vi "Autonomous Independent.vi"   [LabVIEW 2018]
doc: "This VI is called when autonomous begins, and will automatically be terminated when autonomous ends. You can carry out timed or sensor driven robot movement independently without needing to return to the caller."
uses:
  RobotGlobal.vi
  Classes/Pnematics control/Pneumatics.lvclass
  Classes/Pnematics control/Solenoids/Solenoids.lvclass
panel:
  # "Be sure to right-click and choose Data Operations>>Make Current Value default if you want to save the array values with the VI"
types:
  T1 = typedef "RobotObjects.ctl" = cluster{"Drive.lvclass":refnum<class "Drive.lvclass">, "Pneumatics.lvclass":refnum<class "Pneumatics.lvclass">, "Vision.lvclass":refnum<class "Vision.lvclass">, "Joysticks.lvclass":refnum<class "Joysticks.lvclass">, "Elevator.lvclass":refnum<class "Elevator.lvclass">, "Hatch.lvclass":refnum<class "Hatch.lvclass">, "Cargo.lvclass":refnum<class "Cargo.lvclass">}
  T2 = typedef "Pneumatics control.lvlib/Pneumatics.lvclass/Solenoids.ctl" = cluster{"DriveShift":refnum<class "Solenoids.lvclass">, "ArmLock":refnum<class "Solenoids.lvclass">, "HatchArm":refnum<class "Solenoids.lvclass">, "HatchGrabber":refnum<class "Solenoids.lvclass">}
  T3 = cluster{"[0]":refnum<class "Solenoids.lvclass">, "[1]":refnum<class "Solenoids.lvclass">, "[2]":refnum<class "Solenoids.lvclass">, "[3]":refnum<class "Solenoids.lvclass">}
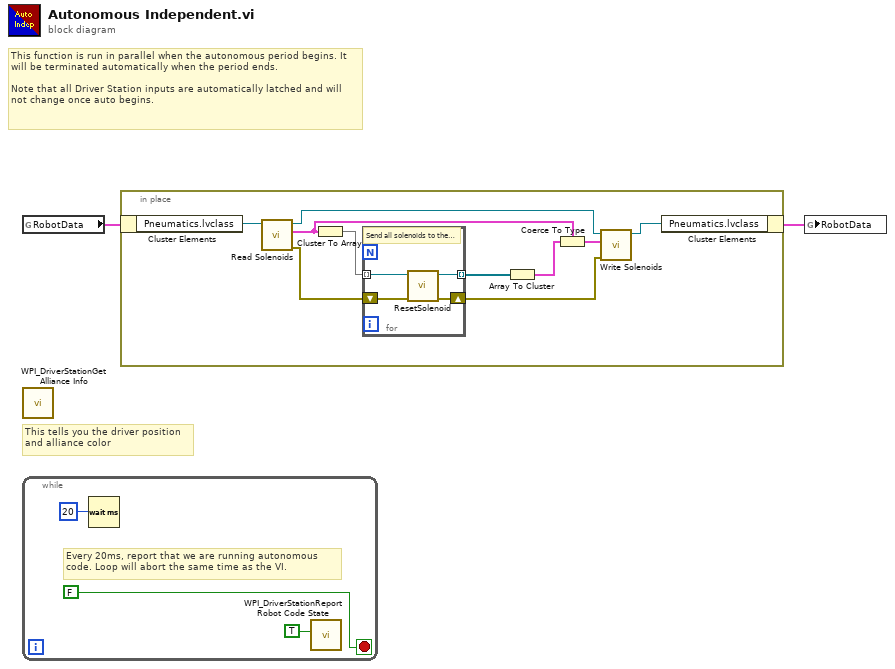
[diagram p0: block diagram]
diagram:
  # "This function is run in parallel when the autonomous period begins. It will be terminated automatically when the period ends.\n\nNote that all Driver Station inputs are automatically latched and will not change once auto begins."
  # "This tells you the driver position\nand alliance color"
  n1 = global read "RobotGlobal.vi" "RobotData"() -> (w2:T1)
  n2 = call <vilib>:"WPI_DriverStationGet Alliance Info.vi"() -> ()  [unwired: 12 out]
  n3 = while {
    stop <- FALSE stop-if-true
    # "Every 20ms, report that we are running autonomous\ncode. Loop will abort the same time as the VI."
    n4 = Wait (ms)(milliseconds to wait=u32 20) -> ()  [unwired: 1 out]
    n5 = call <vilib>:"WPI_DriverStationReport Robot Code State.vi"("Autonomous"=TRUE) -> ()  [unwired: 10 in, 1 out]
  }
  n6 = in-place {
    n7 = in-place-cluster #1(w2) -> ("Pneumatics.lvclass"=w9:refnum<class "Pneumatics.lvclass">)
    n8 = call-dynamic "Read Solenoids.vi"("Pneumatics in"=w9) -> ("error out"=w7:errorcluster, "Solenoids"=w10:T2, "Pneumatics out"=w15:refnum<class "Pneumatics.lvclass">)  [unwired: 8 in]
    n9 = Cluster To Array(cluster=w10) -> (array=w14:refnum<class "Solenoids.lvclass">[])
    n10 = for {
      tunnel: [w19] -> w13 mode=indexing
      tunnel: w14 -> [w18] mode=indexing
      shift-right: [w16] -> w6
      shift-left: w7 -> [w17]
      # "Send all solenoids to the correct position"
      n11 = call-dynamic "ResetSolenoid.vi"("error in (no error)"=w17, "Solenoids in"=w18) -> ("error out"=w16:errorcluster, "Solenoids out"=w19:refnum<class "Solenoids.lvclass">)  [unwired: 8 in]
    }
    n12 = Array To Cluster(array=w13) -> (cluster=w12:T3)
    n13 = Coerce To Type(0:w12, 1:w10) -> (2:w11:T2)
    n14 = call-dynamic "Write Solenoids.vi"("error in (no error)"=w6, "Solenoids"=w11, "Pneumatics in"=w15) -> ("Pneumatics out"=w8:refnum<class "Pneumatics.lvclass">)  [unwired: 7 in, 1 out]
    n15 = in-place-cluster #1("Pneumatics.lvclass"=w8) -> (w1:T1)
  }
  n16 = global write "RobotGlobal.vi" "RobotData"(w1) -> ()
